vi "固定扫码器扫码.vi"(8 "error in (no error)":errorcluster, 11 "VISA资源名称":refnum<visa-resource-name>="COM5") -> (0 "error out":errorcluster, 2 "响应":string)   [LabVIEW 2020]
uses:
  E:/National Instruments/LabVIEW 2018/examples/Instrument IO/Serial/support/Serial - Settings.ctl
  <vilib>/Instr/_visa.llb/VISA Configure Serial Port (Instr).vi
panel:
  in  "串口设置":T1={"波特率"=9600, "数据位"=8, "校验"=enum."None", "停止位"=10, "流控制"=0} {"流控制" items=["无"=0, "XON/XOFF"=1, "RTS/CTS"=2, "DTR/DSR"=4]; "停止位" items=["1.0"=10, "1.5"=15, "2.0"=20]; "数据位" min=5 max=8 step=1; "波特率" items=["75"=75, "110"=110, "134"=134, "150"=150, "300"=300, "600"=600, "1200"=1200, "1800"=1800, "2400"=2400, "4800"=4800, "7200"=7200, "9600"=9600, "14400"=14400, "19200"=19200, "28800"=28800, "38400"=38400, "56000"=56000, "57600"=57600, "115200"=115200, "128000"=128000, "230400"=230400]}
  out "读取的字节":u32
  in  "读取前延时(ms)":u32=3000
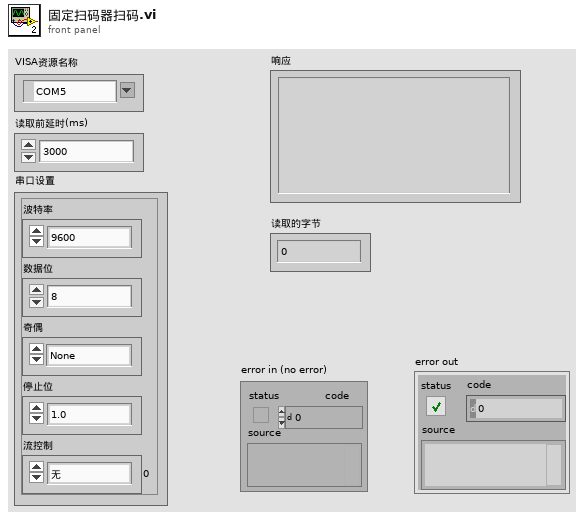
[diagram p1: front panel]
types:
  T1 = typedef "Serial - Settings.ctl" = cluster{"波特率":u32, "数据位":u16, "校验":enum16{"None", "Odd", "Even", "Mark", "Space"}, "停止位":u16, "流控制":u16}
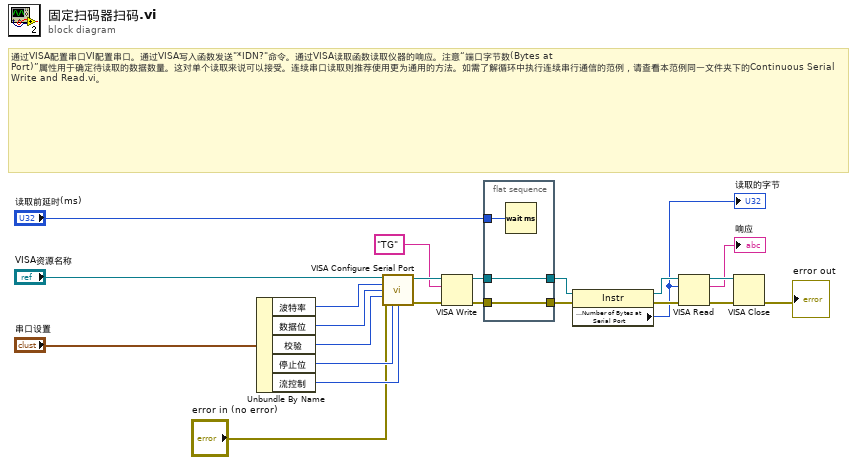
[diagram p0: block diagram]
diagram:
  # "通过VISA配置串口VI配置串口。通过VISA写入函数发送\"*IDN?\"命令。通过VISA读取函数读取仪器的响应。注意“端口字节数(Bytes at Port)”属性用于确定待读取的数据数量。这对单个读取来说可以接受。连续串口读取则推荐使用更为通用的方法。如需了解循环中执行连续串行通信的范例，请查看本范例同一文件夹下的Continuous Serial Write and Read.vi。"
  n1 = Unbundle By Name("串口设置") -> ("波特率"=w6:u32, "数据位"=w5:u16, "校验"=w4:enum16{"None", "Odd", "Even", "Mark", "Space"}, "停止位"=w3:u16, "流控制"=w2:u16)
  n2 = call-poly "VISA Configure Serial Port"("VISA resource name"="VISA资源名称", "baud rate (9600)"=w6, "data bits (8)"=w5, "parity (0:none)"=w4, "error in (no error)"="error in (no error)", "stop bits (10: 1 bit)"=w3, "flow control (0:none)"=w2) -> ("VISA resource name out"=w21:refnum<visa-resource-name>, "error out"=w22:errorcluster)  [unwired: 2 in, 5 out]
  n3 = VISA Write(VISA resource name=w21, write buffer="TG" ("Command"), error in (no error)=w22) -> (VISA resource name out=w15:refnum<visa-resource-name>, error out=w17:errorcluster)  [unwired: 1 out]
  n4 = flat-sequence {
    tunnel: w17 -> [w25]
    tunnel: [w25] -> w16
    tunnel: w15 -> [w24]
    tunnel: [w24] -> w14
    tunnel: "读取前延时(ms)" -> [w26]
    frame #0 {
      n5 = Wait (ms)(milliseconds to wait=w26) -> ()  [unwired: 1 out]
    }
  }
  n6 = property class="Instr"(reference=w14, error in=w16) -> (reference out=w11:refnum<visa-resource-name>, error out=w10:errorcluster, "Serial Settings:Number of Bytes at Serial Port"=w8:u32)
  "读取的字节" <- w8
  n7 = VISA Read(VISA resource name=w11, byte count=w8, error in (no error)=w10) -> (VISA resource name out=w19:refnum<visa-resource-name>, read buffer=→"响应":string, error out=w20:errorcluster)  [unwired: 1 out]
  n8 = VISA Close(VISA resource name=w19, error in (no error)=w20) -> (error out=→"error out":errorcluster)
